vi "ApplyRFdialog_2.vi"(10 "CtlRef":refnum<vi>) -> (0 "drop?":bool, 1 "时钟（分钟） 2":u32=1, 2 "射频出":string(combo)="COM1", 3 "射频进 2":string(combo)="A2")   [LabVIEW 2015]
uses:
  <vilib>/Utility/miscctls.llb/LVComboBoxStrsAndValuesArrayTypeDef.ctl
panel:
  in  "Cancel":bool
  in  "OK":bool
  in  "时间（分钟）":u32=90
  in  "射频进":string(combo)="A1"
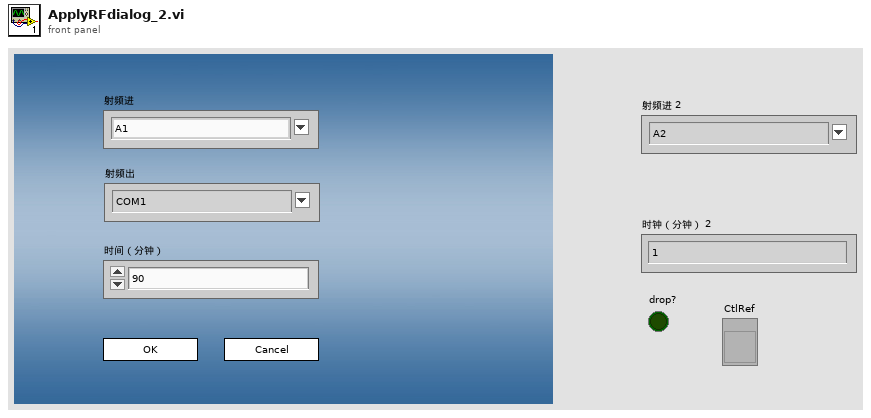
[diagram p1: front panel]
types:
  T1 = typedef "LVComboBoxStrsAndValuesArrayTypeDef.ctl" = cluster{"String":string, "Value":string}[]
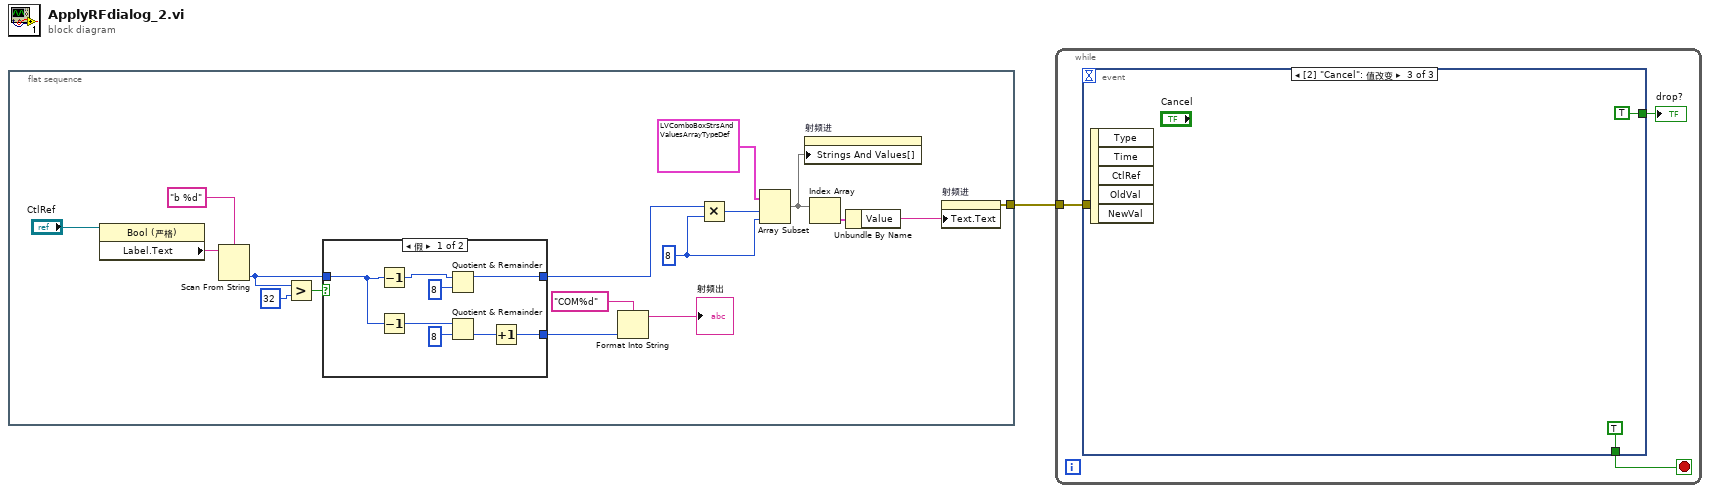
[diagram p0: block diagram]
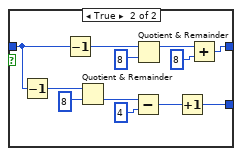
[diagram p2: hidden frame]
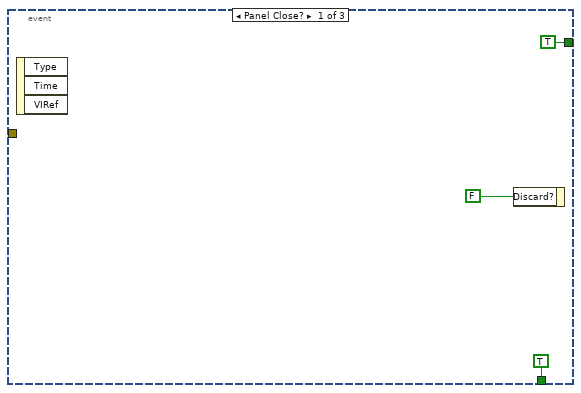
[diagram p3: hidden frame]
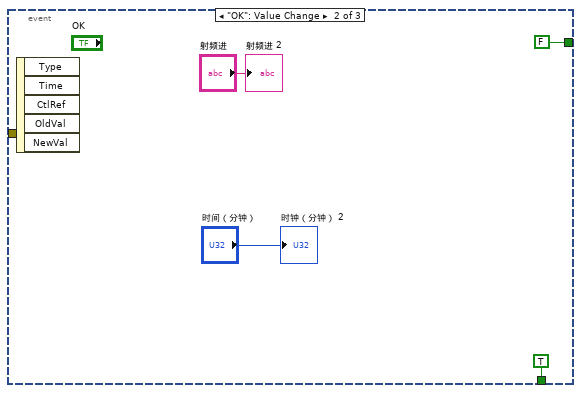
[diagram p4: hidden frame]
diagram:
  n1 = flat-sequence {
    tunnel: [w2] -> w1
    frame #0 {
      w8 = 8 ("length")
      n2 = property class="Bool (严格)"(reference="CtlRef") -> ("Label.Text"=w15:string)  [unwired: 1 in, 2 out]
      n3 = Scan From String(format string="b %d", input string=w15) -> (output 1=w16:i32)  [unwired: 3 in, 3 out]
      n4 = Greater?(x=w16, y=32) -> (0:w18:bool)
      n5 = case shown="假" w18 {
        tunnel: [w23 w27] -> w13
        tunnel: [w19 w34] -> w6
        tunnel: w16 -> [w21 w31]
        frame False {
          n6 = Decrement(x=w21) -> (x-1=w20:i32)
          n7 = Decrement(x=w21) -> (x-1=w26:i32)
          n8 = Quotient & Remainder(x=w20, y=8) -> (x-y*floor(x/y)=w19:i32)  [unwired: 1 out]
          n9 = Quotient & Remainder(x=w26, y=8) -> (floor(x/y)=w24:i32)  [unwired: 1 out]
          n10 = Increment(x=w24) -> (x+1=w23:i32)
        }
        frame True {
          n11 = Decrement(x=w31) -> (x-1=w33:i32)
          n12 = Decrement(x=w31) -> (x-1=w38:i32)
          n13 = Quotient & Remainder(x=w33, y=8) -> (floor(x/y)=w30:i32)  [unwired: 1 out]
          n14 = Subtract(x=w30, y=4) -> (x-y=w28:i32)
          n15 = Quotient & Remainder(x=w38, y=8) -> (x-y*floor(x/y)=w36:i32)  [unwired: 1 out]
          n16 = Increment(x=w28) -> (x+1=w27:i32)
          n17 = Add(x=w36, y=8) -> (x+y=w34:i32)
        }
      }
      n18 = Format Into String(format string="COM%d", w13) -> (resulting string=→"射频出":string)  [unwired: 2 in, 1 out]
      n19 = Multiply(x=w6, y=w8) -> (x*y=w9:i32)
      n20 = Array Subset(array=T1 [{"String"="A1", "Value"="A1"}, {"String"="A2", "Value"="A2"}, {"String"="A3", "Value"="A3"}, {"String"="A4", "Value"="A4"}, {"String"="A5", "Value"="A5"}, {"String"="A6", "Value"="A6"}, {"String"="A7", "Value"="A7"}, {"String"="A8", "Value"="A8"}, {"String"="A9", "Value"="A9"}, {"String"="A10", "Value"="A10"}, {"String"="A11", "Value"="A11"}, {"String"="A12", "Value"="A12"}, {"String"="A13", "Value"="A13"}, {"String"="A14", "Value"="A14"}, {"String"="A15", "Value"="A15"}, {"String"="A16", "Value"="A16"}, {"String"="A17", "Value"="A17"}, {"String"="A18", "Value"="A18"}, {"String"="A19", "Value"="A19"}, {"String"="A20", "Value"="A20"}, {"String"="A21", "Value"="A21"}, {"String"="A22", "Value"="A22"}, {"String"="A23", "Value"="A23"}, {"String"="A24", "Value"="A24"}, {"String"="A25", "Value"="A25"}, {"String"="A26", "Value"="A26"}, {"String"="A27", "Value"="A27"}, {"String"="A28", "Value"="A28"}, {"String"="A29", "Value"="A29"}, {"String"="A30", "Value"="A30"}, {"String"="A31", "Value"="A31"}, {"String"="A32", "Value"="A32"}, {"String"="A33", "Value"="A33"}, {"String"="A34", "Value"="A34"}, {"String"="A35", "Value"="A35"}, {"String"="A36", "Value"="A36"}, {"String"="A37", "Value"="A37"}, {"String"="A38", "Value"="A38"}, {"String"="A39", "Value"="A39"}, {"String"="A40", "Value"="A40"}, {"String"="A41", "Value"="A41"}, {"String"="A42", "Value"="A42"}, {"String"="A43", "Value"="A43"}, {"String"="A44", "Value"="A44"}, {"String"="A45", "Value"="A45"}, {"String"="A46", "Value"="A46"}, {"String"="A47", "Value"="A47"}, {"String"="A48", "Value"="A48"}, {"String"="A49", "Value"="A49"}, {"String"="A50", "Value"="A50"}, {"String"="A51", "Value"="A51"}, {"String"="A52", "Value"="A52"}, {"String"="A53", "Value"="A53"}, {"String"="A54", "Value"="A54"}, {"String"="A55", "Value"="A55"}, {"String"="A56", "Value"="A56"}, {"String"="A57", "Value"="A57"}, {"String"="A58", "Value"="A58"}, {"String"="A59", "Value"="A59"}, {"String"="A60", "Value"="A60"}, {"String"="A61", "Value"="A61"}, {"String"="A62", "Value"="A62"}, {"String"="A63", "Value"="A63"}, {"String"="A64", "Value"="A64"}, {"String"="A65", "Value"="A65"}, {"String"="A66", "Value"="A66"}, {"String"="A67", "Value"="A67"}, {"String"="A68", "Value"="A68"}, {"String"="A69", "Value"="A69"}, {"String"="A70", "Value"="A70"}, {"String"="A71", "Value"="A71"}, {"String"="A72", "Value"="A72"}, {"String"="A73", "Value"="A73"}, {"String"="A74", "Value"="A74"}, {"String"="A75", "Value"="A75"}, {"String"="A76", "Value"="A76"}, {"String"="A77", "Value"="A77"}, {"String"="A78", "Value"="A78"}, {"String"="A79", "Value"="A79"}, {"String"="A80", "Value"="A80"}, {"String"="A81", "Value"="A81"}, {"String"="A82", "Value"="A82"}, {"String"="A83", "Value"="A83"}, {"String"="A84", "Value"="A84"}, {"String"="A85", "Value"="A85"}, {"String"="A86", "Value"="A86"}, {"String"="A87", "Value"="A87"}, {"String"="A88", "Value"="A88"}, {"String"="A89", "Value"="A89"}, {"String"="A90", "Value"="A90"}, {"String"="A91", "Value"="A91"}, {"String"="A92", "Value"="A92"}, {"String"="A93", "Value"="A93"}, {"String"="A94", "Value"="A94"}, {"String"="A95", "Value"="A95"}, {"String"="A96", "Value"="A96"}, {"String"="A97", "Value"="A97"}, {"String"="A98", "Value"="A98"}, {"String"="A99", "Value"="A99"}, {"String"="A100", "Value"="A100"}, {"String"="A101", "Value"="A101"}, {"String"="A102", "Value"="A102"}, {"String"="A103", "Value"="A103"}, {"String"="A104", "Value"="A104"}, {"String"="A105", "Value"="A105"}, {"String"="A106", "Value"="A106"}, {"String"="A107", "Value"="A107"}, {"String"="A108", "Value"="A108"}, {"String"="A109", "Value"="A109"}, {"String"="A110", "Value"="A110"}, {"String"="A111", "Value"="A111"}, {"String"="A112", "Value"="A112"}, {"String"="A113", "Value"="A113"}, {"String"="A114", "Value"="A114"}, {"String"="A115", "Value"="A115"}, {"String"="A116", "Value"="A116"}, {"String"="A117", "Value"="A117"}, {"String"="A118", "Value"="A118"}, {"String"="A119", "Value"="A119"}, {"String"="A120", "Value"="A120"}, {"String"="A121", "Value"="A121"}, {"String"="A122", "Value"="A122"}, {"String"="A123", "Value"="A123"}, {"String"="A124", "Value"="A124"}, {"String"="A125", "Value"="A125"}, {"String"="A126", "Value"="A126"}, {"String"="A127", "Value"="A127"}, {"String"="A128", "Value"="A128"}] ("Strings And Values []"), index=w9, length=w8) -> (w4:T1)
      n21 = property on="射频进" class="CmbBox"("Strings And Values[]"=w4) -> ()  [unwired: 2 in, 2 out]
      n22 = Index Array(array=w4) -> (element=w7:cluster{"String":string, "Value":string})  [unwired: 1 in]
      n23 = Unbundle By Name(w7) -> ("Value"=w3:string)
      n24 = property on="射频进" class="CmbBox"("Text.Text"=w3) -> (error out=w2:errorcluster)  [unwired: 2 in, 1 out]
    }
  }
  n25 = while {
    tunnel: w1 -> [w39]
    stop <- w40 stop-if-true
    n26 = event shown="[2] \"Cancel\": 值改变" {
      selector: _ -> [_ _ _]
      dyn-events: _ -> [_ _ _]
      timeout: _ -> [_ _ _]
      tunnel: [TRUE FALSE TRUE] -> w41
      tunnel: [TRUE TRUE TRUE] -> w40
      tunnel: w39 -> [_ _ _]
      event Panel Close? {
        n27 = event-data() -> ()  [unwired: 1 in, 3 out]
        n28 = event-data("Discard?"=FALSE ("放弃？")) -> ()  [unwired: 1 in, 1 out]
      }
      event "OK": Value Change {
        n29 = event-data() -> ()  [unwired: 1 in, 5 out]
        "射频进 2" <- "射频进"
        "时钟（分钟） 2" <- "时间（分钟）"
      }
      event "Cancel": Value Change {
        n30 = event-data() -> ()  [unwired: 1 in, 5 out]
      }
    }
    "drop?" <- w41
  }
